vi "Get Array Control Size.vi"(8 "error in (no error)":errorcluster, 11 "Array in":refnum<vi>) -> (0 "error out":errorcluster, 2 "Size":i32, 3 "Array out":refnum<vi>)   [LabVIEW 2020, in "UI Common.lvlib"]
uses:
  UI Common.lvlib
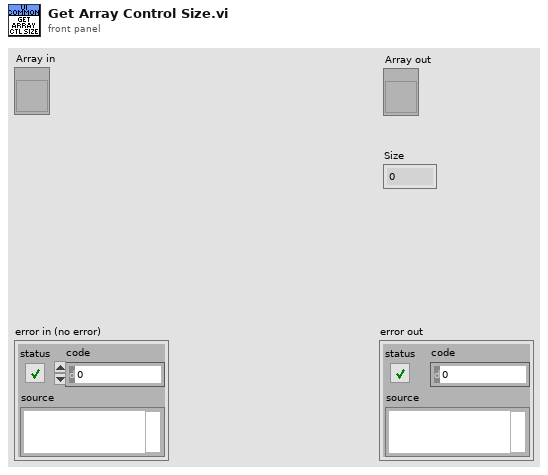
[diagram p1: front panel]
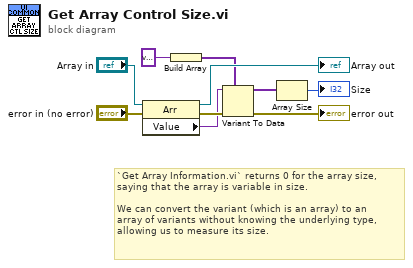
[diagram p0: block diagram]
diagram:
  # "`Get Array Information.vi` returns 0 for the array size,\nsaying that the array is variable in size.\n\nWe can convert the variant (which is an array) to an\narray of variants without knowing the underlying type,\nallowing us to measure its size."
  n1 = property class="Arr"(reference="Array in", error in="error in (no error)") -> (reference out=→"Array out":refnum<vi>, error out=w7:errorcluster, "Value"=w6:variant)
  n2 = Build Array(variant ("Value")) -> (w1:variant[])
  n3 = Variant To Data(error in=w7, type=w1, Variant=w6) -> (data=w2:variant[], error out=→"error out":errorcluster)
  n4 = Array Size(array=w2) -> (size(s)=→"Size":i32)
